vi "AG34980A_DAC_Output_State.vi"(0 "VISA resource name":refnum<visa-resource-name>, 1 "Channel List":string, 7 "Output State (F:Off)":bool, 11 "error in (no error)":errorcluster) -> (4 "VISA resource name out":refnum<visa-resource-name>, 15 "error out":errorcluster)   [LabVIEW 2019]
doc: "This VI disables or enables the output state of the specified channels on the 34951A Isolated DAC Module. When enabled, the corresponding output relay is closed thus enabling signal outputs from the specified channels."
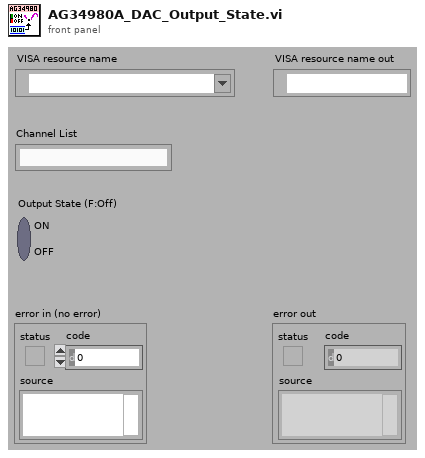
[diagram p1: front panel]
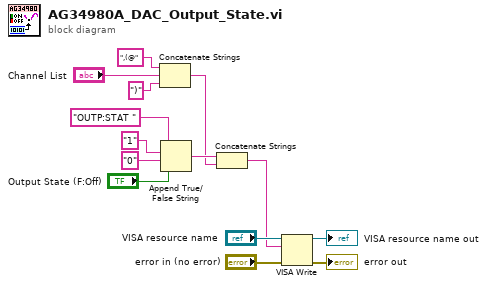
[diagram p0: block diagram]
diagram:
  n1 = Concatenate Strings(",(@", "Channel List", ")") -> (w2:string)
  n2 = Append True/False String(1:"Output State (F:Off)", 2:"0" ("false string"), 3:"1" ("true string"), 4:"OUTP:STAT " ("string (\"\")")) -> (0:w3:string)
  n3 = Concatenate Strings(w3, w2) -> (w1:string)
  n4 = VISA Write(VISA resource name="VISA resource name", write buffer=w1, error in (no error)="error in (no error)") -> (VISA resource name out=→"VISA resource name out":refnum<visa-resource-name>, error out=→"error out":errorcluster)  [unwired: 1 out]
